vi "FPGAPowerMeasurement4withoutTrigger.vi"() -> ()   [LabVIEW 2009]
uses:
  <vilib>/express/express analysis/Spectral/XNode/ExpressSpectralMeasurementsBlockNode.xnode
  <vilib>/express/express analysis/Spectral/Block/exnSpectralBlock spectral measurements PSD poly.vi
  <vilib>/express/express analysis/Spectral/Block/exnSpectralBlock spectral measurements PSD DDT.vi
panel:
  out "Temperature":dynamicdata(graph)
  out "Waveform Graph 3":dynamicdata(graph)
  out "Waveform Graph 2":dynamicdata(graph)
  out "Waveform Graph":dynamicdata(graph)
  out "Voltage at FPGA":dynamicdata(graph)
  out "Power":dynamicdata(graph)
  out "Average Power":dbl
  out "Average Voltage":dbl
  out "Average Current":dbl
  out "Current":dynamicdata(graph)
  in  "stop":bool
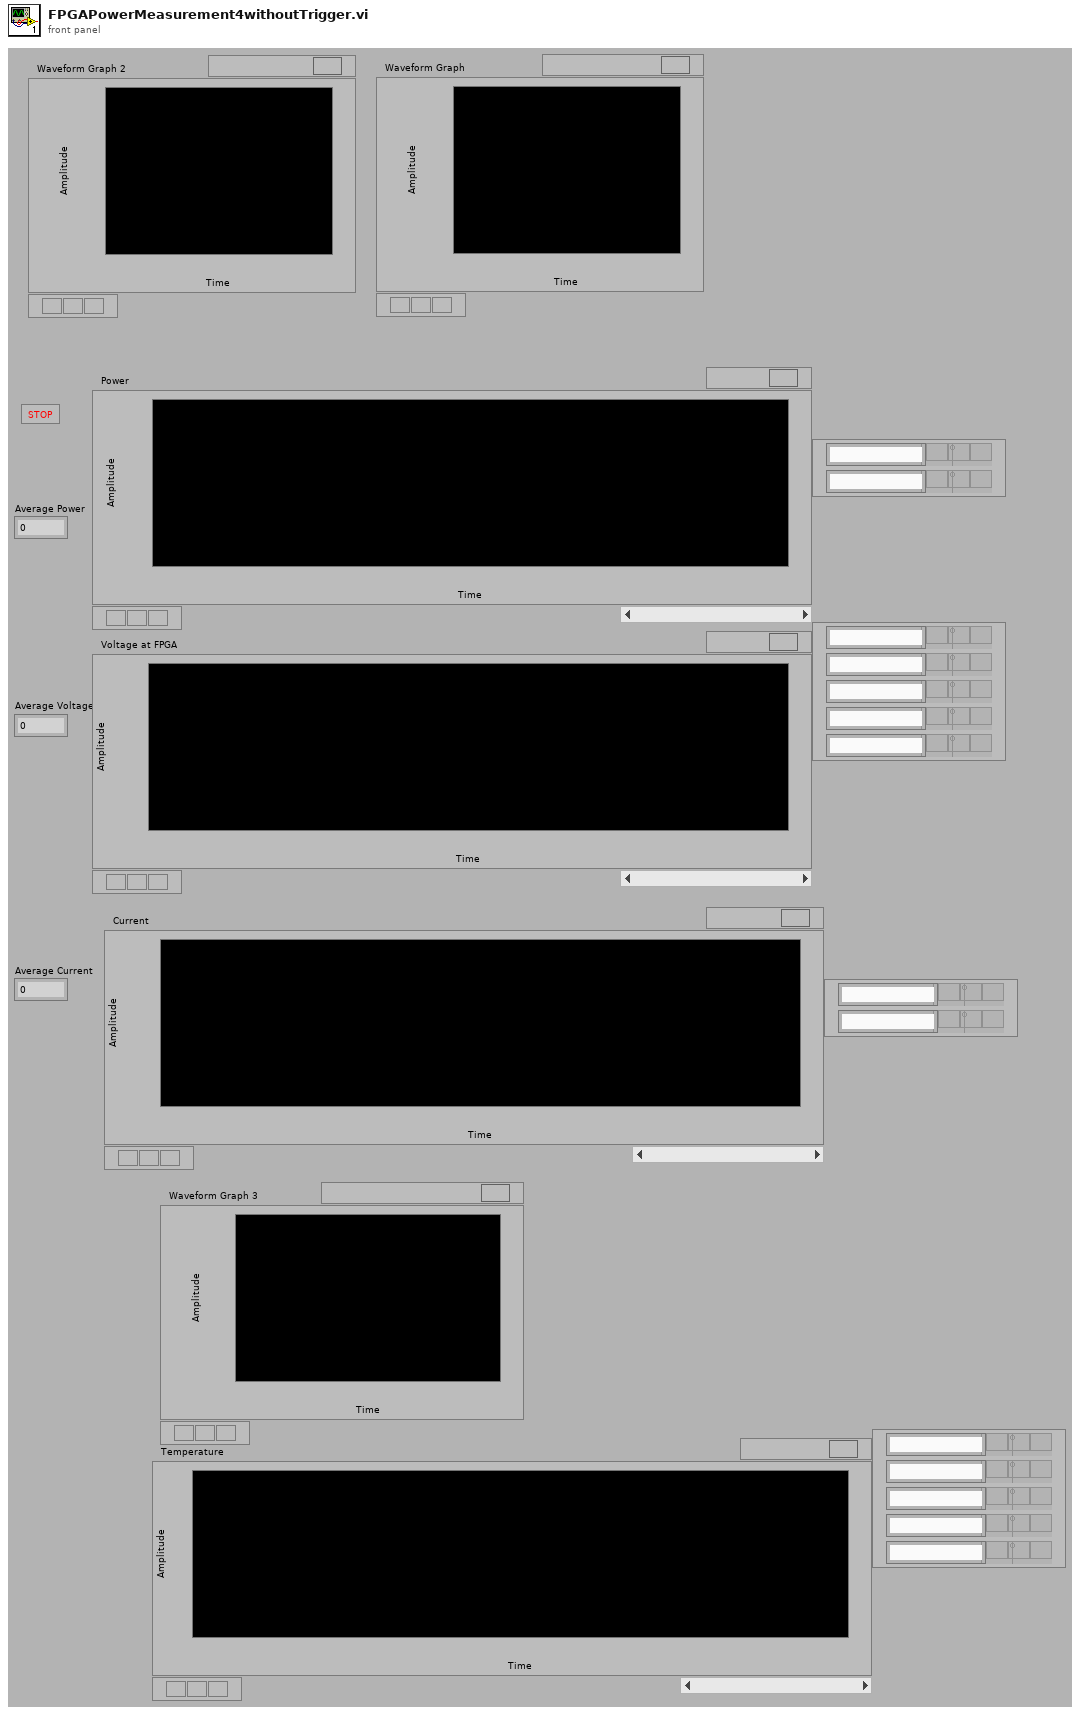
[diagram p1: front panel]
types:
  T1 = typedef "LVTextColorsTypeDef.ctl" = cluster{"Text Color":u32, "Background Color":u32}
  T2 = typedef "LVRangeTypeDef.ctl" = cluster{"Minimum":dbl, "Maximum":dbl, "Increment":dbl, "Minor Increment":dbl, "Start":dbl}
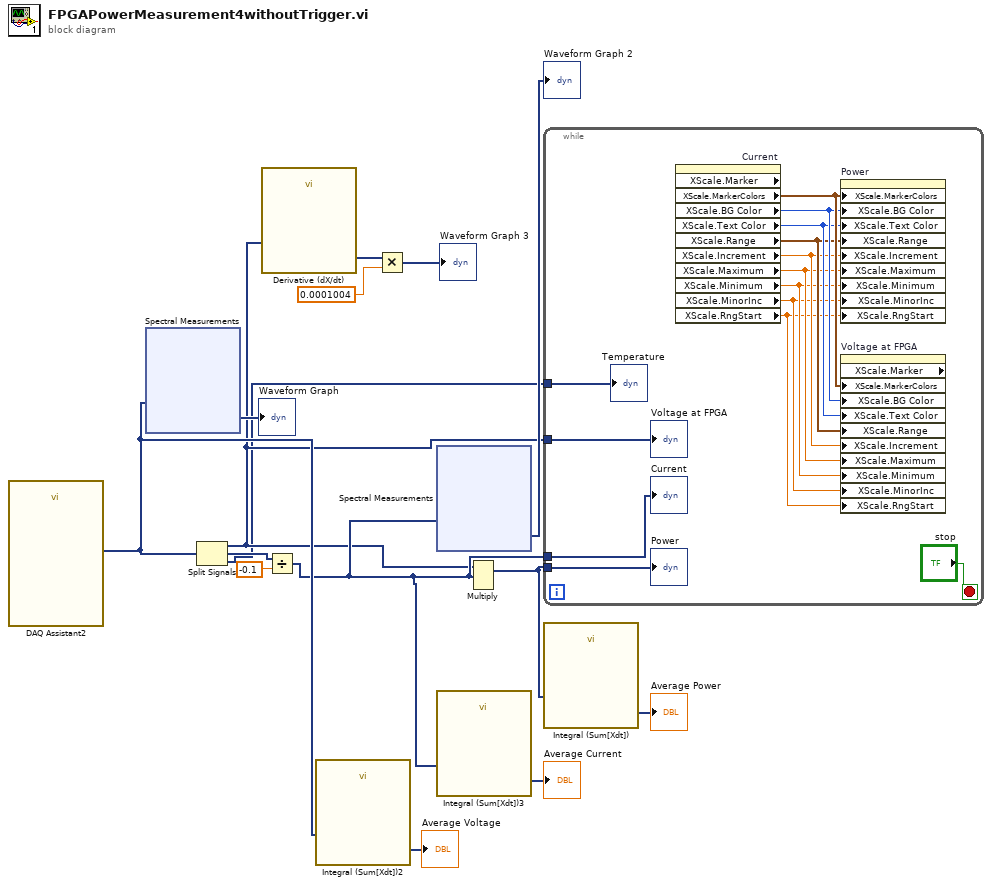
[diagram p0: block diagram]
diagram:
  n1 = call "DAQ Assistant2"() -> ("data"=w4:dynamicdata)  [unwired: 17 in, 2 out]
  n2 = xnode "Spectral Measurements"("Signals"=w4) -> ("PSD"=→"Waveform Graph":dynamicdata)  [unwired: 1 in, 1 out]
  n3 = Split Signals(w4) -> (w2:dynamicdata, w5:dynamicdata, w1:dynamicdata)  [unwired: 3 in]
  n4 = call "Derivative (dX/dt)"("Signals"=w2) -> ("Result"=w8:dynamicdata)  [unwired: 5 in, 1 out]
  n5 = Divide(x=w5, y=-0.1) -> (x/y=w3:dynamicdata)
  n6 = call "Integral (Sum[Xdt])2"("Signals"=w4) -> ("Result"=→"Average Voltage":dynamicdata)  [unwired: 5 in, 1 out]
  n7 = Multiply(x=w8, y=0.0001004) -> (x*y=→"Waveform Graph 3":dynamicdata)
  n8 = xnode "Spectral Measurements"("Signals"=w3) -> ("PSD"=→"Waveform Graph 2":dynamicdata)  [unwired: 1 in, 1 out]
  n9 = call "Integral (Sum[Xdt])3"("Signals"=w3) -> ("Result"=→"Average Current":dynamicdata)  [unwired: 5 in, 1 out]
  n10 = Multiply(1:w3, 2:w2) -> (0:w15:dynamicdata)  [unwired: 1 in, 1 out]
  n11 = while {
    tunnel: w15 -> [w28]
    tunnel: w3 -> [w18]
    tunnel: w2 -> [w17]
    tunnel: w1 -> [w16]
    stop <- "stop" stop-if-true
    n12 = property on="Current" class="WFGraph (strict)" props=["XScale", "Marker", "XScale", "MarkerColors", "XScale", "BG Color", "XScale", "Text Color", "XScale", "Range", "XScale", "Increment", "XScale", "Maximum", "XScale", "Minimum", "XScale", "MinorInc", "XScale", "RngStart"]() -> ("XScale.MarkerColors"=w27:T1, "XScale.BG Color"=w26:u32, "XScale.Text Color"=w25:u32, "XScale.Range"=w24:T2, "XScale.Increment"=w23:dbl, "XScale.Maximum"=w22:dbl, "XScale.Minimum"=w21:dbl, "XScale.MinorInc"=w20:dbl, "XScale.RngStart"=w19:dbl)  [unwired: 2 in, 3 out]
    n13 = property on="Power" class="WFGraph (strict)"("XScale.MarkerColors"=w27, "XScale.BG Color"=w26, "XScale.Text Color"=w25, "XScale.Range"=w24, "XScale.Increment"=w23, "XScale.Maximum"=w22, "XScale.Minimum"=w21, "XScale.MinorInc"=w20, "XScale.RngStart"=w19) -> ()  [unwired: 2 in, 2 out]
    n14 = property on="Voltage at FPGA" class="WFGraph (strict)" props=["XScale", "Marker", "XScale", "MarkerColors", "XScale", "BG Color", "XScale", "Text Color", "XScale", "Range", "XScale", "Increment", "XScale", "Maximum", "XScale", "Minimum", "XScale", "MinorInc", "XScale", "RngStart"]("XScale.MarkerColors"=w27, "XScale.BG Color"=w26, "XScale.Text Color"=w25, "XScale.Range"=w24, "XScale.Increment"=w23, "XScale.Maximum"=w22, "XScale.Minimum"=w21, "XScale.MinorInc"=w20, "XScale.RngStart"=w19) -> ()  [unwired: 2 in, 3 out]
    "Current" <- w18
    "Power" <- w28
    "Voltage at FPGA" <- w17
    "Temperature" <- w16
  }
  n15 = call "Integral (Sum[Xdt])"("Signals"=w15) -> ("Result"=→"Average Power":dynamicdata)  [unwired: 5 in, 1 out]
